vi "CreateZernikeArray.vi"(10 "General settings":T1) -> (0 "Mode IDs":string[](array[string]), 3 "Modes Out":dbl[][][](array[numeric]))   [LabVIEW 2014]
uses:
  Controls/SLM General Settings.ctl
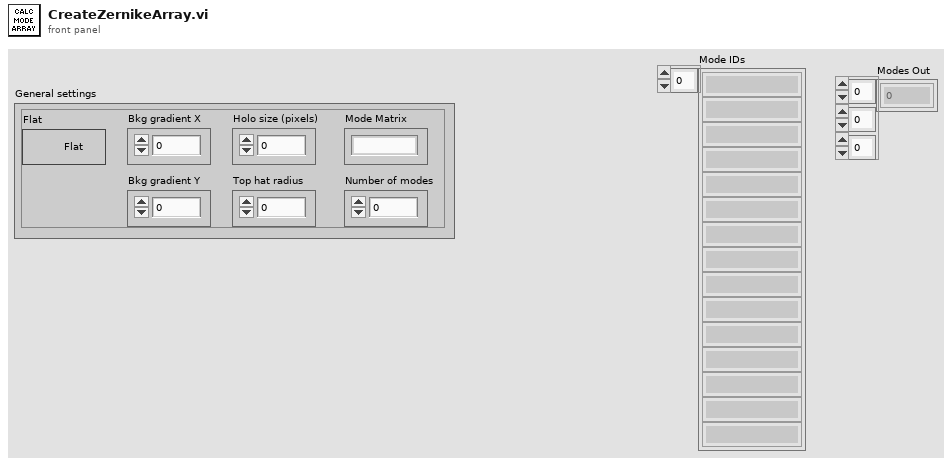
[diagram p1: front panel]
types:
  T1 = typedef "SLM General Settings.ctl" = cluster{"Holo size (pixels)":i32, "Top hat radius":dbl, "Number of modes":i32, "Bkg gradient X":dbl, "Bkg gradient Y":dbl, "Flat":bool, "Mode Matrix":u16}
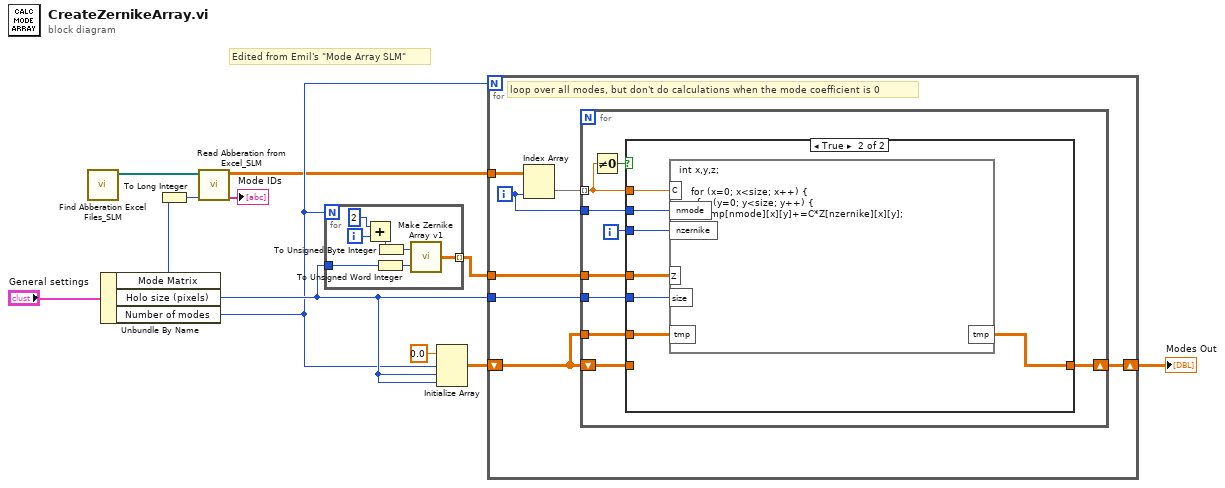
[diagram p0: block diagram]
diagram:
  # "Edited from Emil's \"Mode Array SLM\""
  n1 = call "Find Abberation Excel Files_SLM.vi"() -> ("Abberation File Paths"=w1:path[])  [unwired: 10 in, 1 out]
  n2 = Unbundle By Name("General settings") -> ("Mode Matrix"=w4:u16, "Holo size (pixels)"=w8:i32, "Number of modes"=w7:i32)
  n3 = To Long Integer(number=w4) -> (32bit integer=w2:i32)
  n4 = call "Read Abberation from Excel_SLM.vi"("index"=w2, "Mode Matrices"=w1) -> ("Mode IDs"=→"Mode IDs":string[], "Mode"=w5:dbl[][])  [unwired: 6 in]
  n5 = for {
    N: w7 -> [_]
    tunnel: w8 -> [w19]
    tunnel: [w15] -> w9 mode=indexing
    i -> [w17]
    n6 = Add(x=2, y=w17) -> (x+y=w18:i32)
    n7 = To Unsigned Word Integer(number=w19) -> (unsigned 16bit integer=w14:u16)
    n8 = To Unsigned Byte Integer(number=w18) -> (unsigned 8bit integer=w13:u8)
    n9 = call "Make Zernike Array v1.vi"("size"=w14, "z"=w13) -> ("zernike array"=w15:dbl[][])
  }
  n10 = Initialize Array(0.0 ("element"), w7, w8, w8) -> (w11:dbl[][][])
  n11 = for {
    N: w7 -> [_]
    tunnel: w5 -> [w25]
    tunnel: w8 -> [w24]
    tunnel: w9 -> [w23]
    shift-right: [w20] -> w6
    shift-left: w11 -> [w22]
    i -> [w21]
    # "loop over all modes, but don't do calculations when the mode coefficient is 0"
    n12 = Index Array(array=w25, index (col)=w21) -> (element=w26:dbl[])  [unwired: 1 in]
    n13 = for {
      shift-right: [w28] -> w20
      shift-left: w22 -> [w29]
      tunnel: w23 -> [w32]
      tunnel: w24 -> [w35]
      tunnel: w26 -> [w31] mode=indexing
      tunnel: w22 -> [w34]
      tunnel: w21 -> [w27]
      i -> [w33]
      n14 = Not Equal To 0?(x=w31) -> (x != 0?=w30:bool)
      n15 = case shown="True" w30 {
        tunnel: w35 -> [_ w43]
        tunnel: w34 -> [_ w42]
        tunnel: w31 -> [_ w41]
        tunnel: w33 -> [_ w40]
        tunnel: w32 -> [_ w39]
        tunnel: w29 -> [w36 _]
        tunnel: [w36 w37] -> w28
        tunnel: w27 -> [_ w38]
        frame False {
        }
        frame True {
          n16 = formula code="int x,y,z;\n\n    for (x=0; x<size; x++) {\n      for (y=0; y<size; y++) {\n         tmp[nmode][x][y]+=C*Z[nzernike][x][y];\n      }\n   }"("C"=w41, "size"=w43, "tmp"=w42, "nzernike"=w40, "Z"=w39, "nmode"=w38) -> ("tmp"=w37:dbl[][][])
        }
      }
    }
  }
  "Modes Out" <- w6
